vi "Setup.vi"(8 "error in (no error)":errorcluster, 11 "KST101 in":refnum<class "KST101.lvclass">) -> (0 "error out":errorcluster, 3 "KST101 out":refnum<class "KST101.lvclass">)   [LabVIEW 2016, in "Stepper Motor Controller.lvlib" / "KST101.lvclass"]
uses:
  KST101.lvclass
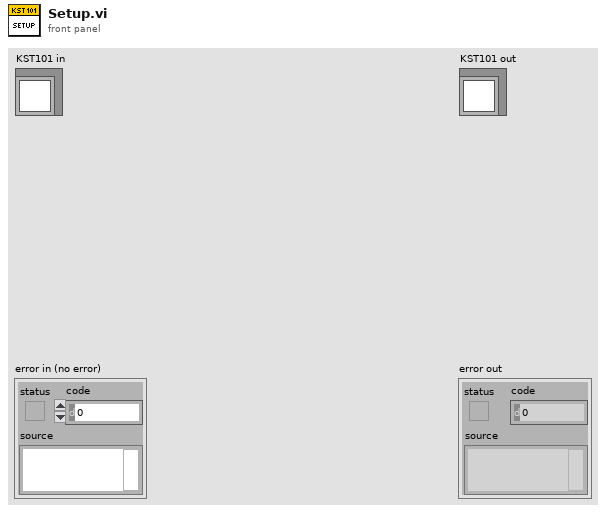
[diagram p1: front panel]
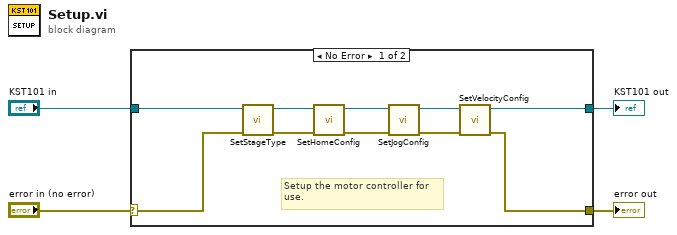
[diagram p0: block diagram]
diagram:
  n1 = case shown="No Error" "error in (no error)" {
    selector: "error in (no error)" -> [w7 w16]
    tunnel: [w9 w16] -> w3
    tunnel: [w12 w15] -> w1
    tunnel: "KST101 in" -> [w8 w15]
    frame No Error {
      # "Setup the motor controller for\nuse."
      n2 = call-dynamic "SetStageType.vi"("error in (no error)"=w7, "KST101 in"=w8) -> ("error out"=w5:errorcluster, "KST101 out"=w6:refnum<class "KST101.lvclass">)  [unwired: 8 in]
      n3 = call-dynamic "SetHomeConfig.vi"("error in (no error)"=w5, "KST101 in"=w6) -> ("error out"=w11:errorcluster, "KST101 out"=w14:refnum<class "KST101.lvclass">)  [unwired: 8 in]
      n4 = call-dynamic "SetJogConfig.vi"("error in (no error)"=w11, "KST101 in"=w14) -> ("error out"=w10:errorcluster, "KST101 out"=w13:refnum<class "KST101.lvclass">)  [unwired: 8 in]
      n5 = call-dynamic "SetVelocityConfig.vi"("error in (no error)"=w10, "KST101 in"=w13) -> ("error out"=w9:errorcluster, "KST101 out"=w12:refnum<class "KST101.lvclass">)  [unwired: 8 in]
    }
    frame Error {
    }
  }
  "error out" <- w3
  "KST101 out" <- w1
